vi "Potentiometer Control.vi"(0 "Arm Window Axis":dbl, 5 "Potentiometer Input":dbl, 7 "Max/Min/Settings Cluster":T2, 9 "Boolean Cluster":T1) -> (6 "Output Motor Speed":dbl)   [LabVIEW 2014]
uses:
  Robot Global Data.vi
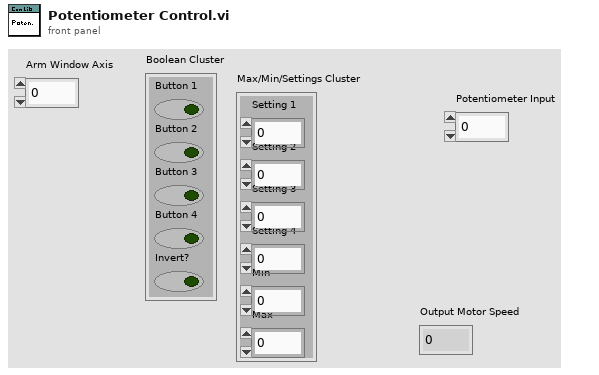
[diagram p1: front panel]
types:
  T1 = cluster{"Button 1":bool, "Button 2":bool, "Button 3":bool, "Button 4":bool, "Invert?":bool}
  T2 = cluster{"Setting 1":dbl, "Setting 2":dbl, "Setting 3":dbl, "Setting 4":dbl, "Min":dbl, "Max":dbl}
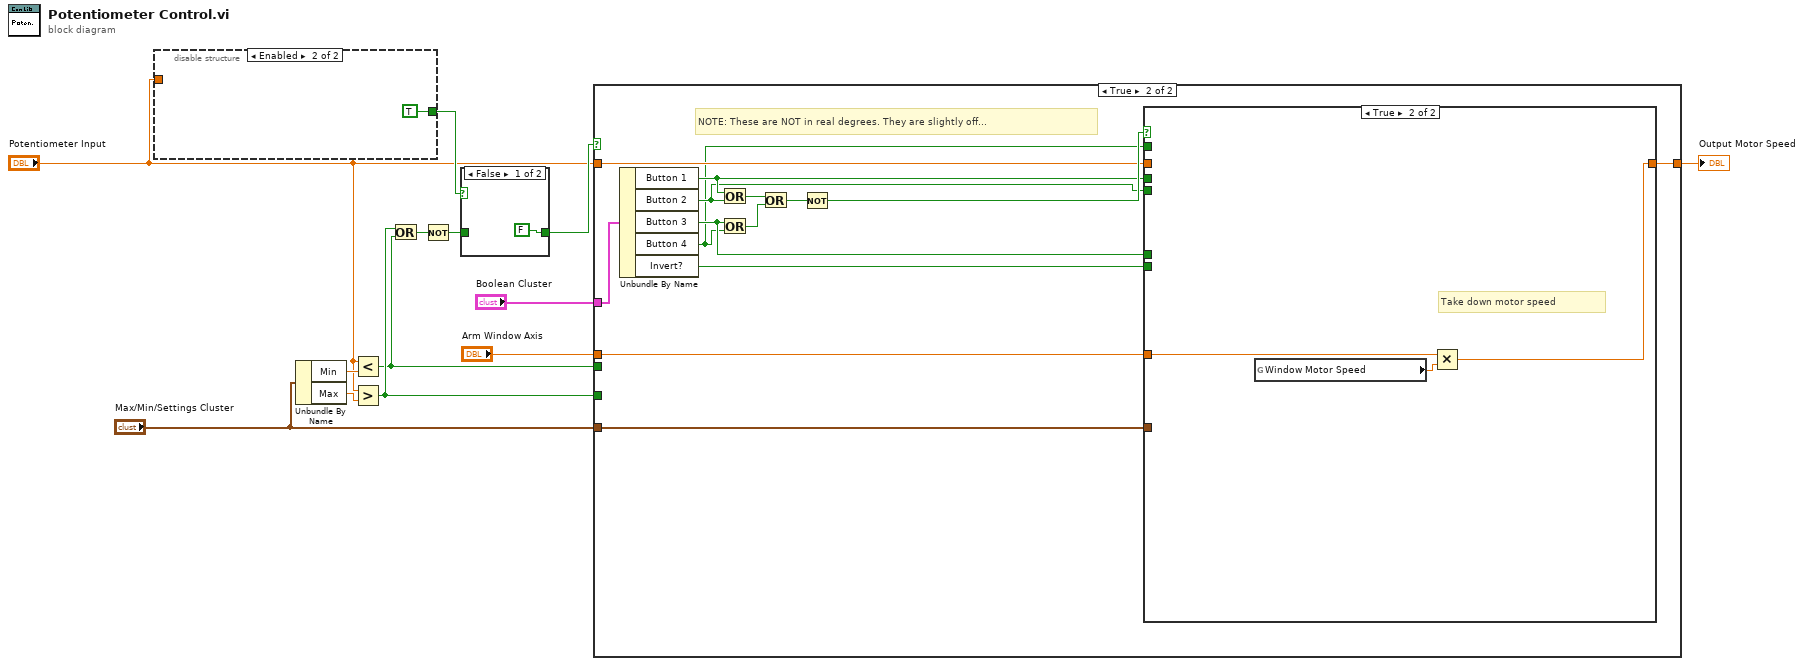
[diagram p0: block diagram]
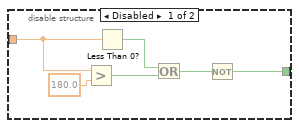
[diagram p2: hidden frame]
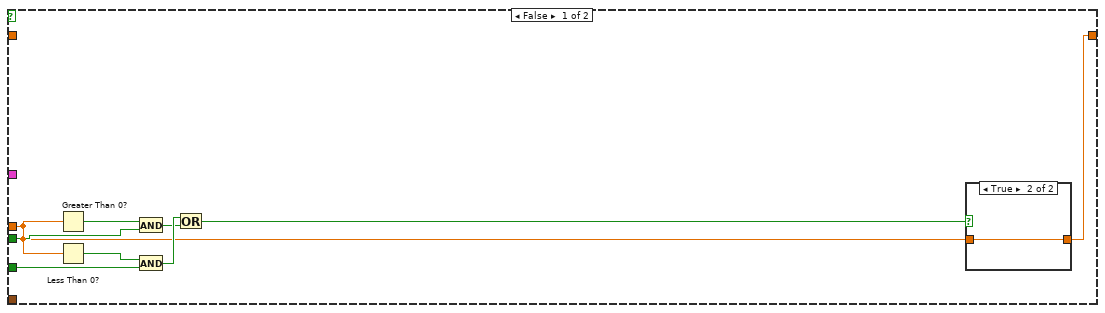
[diagram p4: hidden frame]
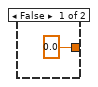
[diagram p5: hidden frame]
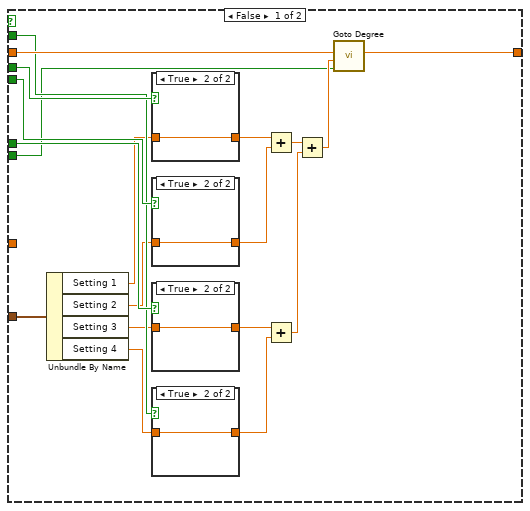
[diagram p6: hidden frame]
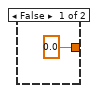
[diagram p7: hidden frame]
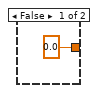
[diagram p8: hidden frame]
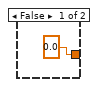
[diagram p9: hidden frame]
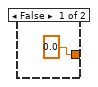
[diagram p10: hidden frame]
diagram:
  n1 = disable-structure shown="Enabled" {
    disable-tunnel: "Potentiometer Input" -> [w18 _]
    disable-tunnel: [w14 TRUE] -> w7
    frame Disabled {
      n2 = Greater?(x=w18, y=180.0) -> (0:w16:bool)
      n3 = Less Than 0?(x=w18) -> (x < 0?=w19:bool)
      n4 = Or(x=w19, y=w16) -> (x .or. y?=w15:bool)
      n5 = Not(x=w15) -> (.not. x?=w14:bool)
    }
    frame Enabled {
    }
  }
  n6 = Unbundle By Name("Max/Min/Settings Cluster") -> ("Min"=w11:dbl, "Max"=w12:dbl)
  n7 = Less?(x="Potentiometer Input", y=w11) -> (x < y?=w1:bool)
  n8 = Greater?(x="Potentiometer Input", y=w12) -> (0:w2:bool)
  n9 = Or(x=w2, y=w1) -> (x .or. y?=w13:bool)
  n10 = Not(x=w13) -> (.not. x?=w8:bool)
  n11 = case shown="False" w7 {
    tunnel: [FALSE w22] -> w9
    tunnel: w8 -> [_ w22]
    frame False {
    }
    frame True {
    }
  }
  n12 = case shown="True" w9 {
    tunnel: "Potentiometer Input" -> [_ w43]
    tunnel: "Max/Min/Settings Cluster" -> [_ w42]
    tunnel: "Boolean Cluster" -> [_ w41]
    tunnel: [w25 w35] -> w4
    tunnel: "Arm Window Axis" -> [w24 w34]
    tunnel: w2 -> [w30 _]
    tunnel: w1 -> [w26 _]
    frame False {
      n13 = Greater Than 0?(x=w24) -> (x > 0?=w27:bool)
      n14 = Less Than 0?(x=w24) -> (x < 0?=w31:bool)
      n15 = And(x=w27, y=w26) -> (x .and. y?=w28:bool)
      n16 = And(x=w31, y=w30) -> (x .and. y?=w29:bool)
      n17 = Or(x=w29, y=w28) -> (x .or. y?=w23:bool)
      n18 = case shown="True" w23 {
        tunnel: [0.0 w33] -> w25
        tunnel: w24 -> [_ w33]
        frame False {
        }
        frame True {
        }
      }
    }
    frame True {
      # "NOTE: These are NOT in real degrees. They are slightly off..."
      n19 = Unbundle By Name(w41) -> ("Button 1"=w40:bool, "Button 2"=w39:bool, "Button 3"=w38:bool, "Button 4"=w37:bool, "Invert?"=w36:bool)
      n20 = Or(x=w40, y=w39) -> (x .or. y?=w45:bool)
      n21 = Or(x=w38, y=w37) -> (x .or. y?=w46:bool)
      n22 = Or(x=w45, y=w46) -> (x .or. y?=w44:bool)
      n23 = Not(x=w44) -> (.not. x?=w47:bool)
      n24 = case shown="True" w47 {
        tunnel: w34 -> [_ w77]
        tunnel: w43 -> [w66 _]
        tunnel: [w65 w76] -> w35
        tunnel: w40 -> [w57 _]
        tunnel: w39 -> [w56 _]
        tunnel: w38 -> [w55 _]
        tunnel: w37 -> [w54 _]
        tunnel: w36 -> [w53 _]
        tunnel: w42 -> [w52 _]
        frame False {
          n25 = Unbundle By Name(w52) -> ("Setting 1"=w51:dbl, "Setting 2"=w50:dbl, "Setting 3"=w49:dbl, "Setting 4"=w48:dbl)
          n26 = case shown="True" w57 {
            tunnel: [0.0 w74] -> w61
            tunnel: w51 -> [_ w74]
            frame False {
            }
            frame True {
            }
          }
          n27 = case shown="True" w56 {
            tunnel: [0.0 w72] -> w62
            tunnel: w50 -> [_ w72]
            frame False {
            }
            frame True {
            }
          }
          n28 = case shown="True" w55 {
            tunnel: [0.0 w70] -> w60
            tunnel: w49 -> [_ w70]
            frame False {
            }
            frame True {
            }
          }
          n29 = case shown="True" w54 {
            tunnel: [0.0 w68] -> w59
            tunnel: w48 -> [_ w68]
            frame False {
            }
            frame True {
            }
          }
          n30 = Add(x=w61, y=w62) -> (x+y=w63:dbl)
          n31 = Add(x=w60, y=w59) -> (x+y=w58:dbl)
          n32 = Add(x=w63, y=w58) -> (x+y=w64:dbl)
          n33 = call "Goto Degree.vi"("Invert Motor"=w53, "Target Degrees"=w64, "Input Degrees"=w66) -> ("Output Motor Speed"=w65:dbl)  [unwired: 8 in]
        }
        frame True {
          # "Take down motor speed"
          n34 = global read "Robot Global Data.vi" "Window Motor Speed"() -> (w75:dbl)
          n35 = Multiply(x=w77, y=w75) -> (x*y=w76:dbl)
        }
      }
    }
  }
  "Output Motor Speed" <- w4
